vi "RS_SMBV100A_N_ASKCONFIGURATION.vi"(0 "DriverConnect in":T2={"InterfaceType"=enum."VISA", "OpenedSession"="", "InterfaceSettings"={"Interface"=enum."RS232", "EOS 4 read"=enum."LF (\\n)", "EOS 4 write"=enum."LF (\\n)", "TMO, ms"=10000, "Sett"=variant(cluster{"Baud Rate":u32, "Data Bits":u16, "Parity":u16, "Stop Bits":u16, "Flow Control":u16, "Eho":bool} {"Baud Rate"=75, "Data Bits"=0, "Parity"=0, "Stop Bits"=0, "Flow Control"=0, "Eho"=FALSE})}}, 1 "BASEBAND":string, 2 "mass":string, 9 "Error In":errorcluster) -> (3 "wrong sat":bool, 4 "DriverConnect out":T2={"InterfaceType"=enum."VISA", "OpenedSession"="", "InterfaceSettings"={"Interface"=enum."RS232", "EOS 4 read"=enum."LF (\\n)", "EOS 4 write"=enum."LF (\\n)", "TMO, ms"=10000, "Sett"=variant(cluster{"Baud Rate":u32, "Data Bits":u16, "Parity":u16, "Stop Bits":u16, "Flow Control":u16, "Eho":bool} {"Baud Rate"=75, "Data Bits"=0, "Parity"=0, "Stop Bits"=0, "Flow Control"=0, "Eho"=FALSE})}}, 6 "Parsing Satelite":T1, 10 "Error Out":errorcluster)   [LabVIEW 2018]
uses:
  MOKO_LabViewLibrary/MokoLowLevel/MokoLowLovelControl/MLLC_ConnectCluster.ctl
  MOKO_LabViewLibrary/MokoLowLevel/MokoLowLovelControl/MLLC_InterfaceType.ctl
  MOKO_LabViewLibrary/MokoLowLevel/MokoLowLovelControl/MLLC_OpenedSession.ctl
  MOKO_LabViewLibrary/MokoLowLevel/MokoLowLovelControl/MLLC_InterfaceSettings.ctl
  MOKO_LabViewLibrary/MokoLowLevel/MokoLowLovelControl/MLLC_InterfaceKind.ctl
  RS_SMBV100A_Parsing Satelite.ctl
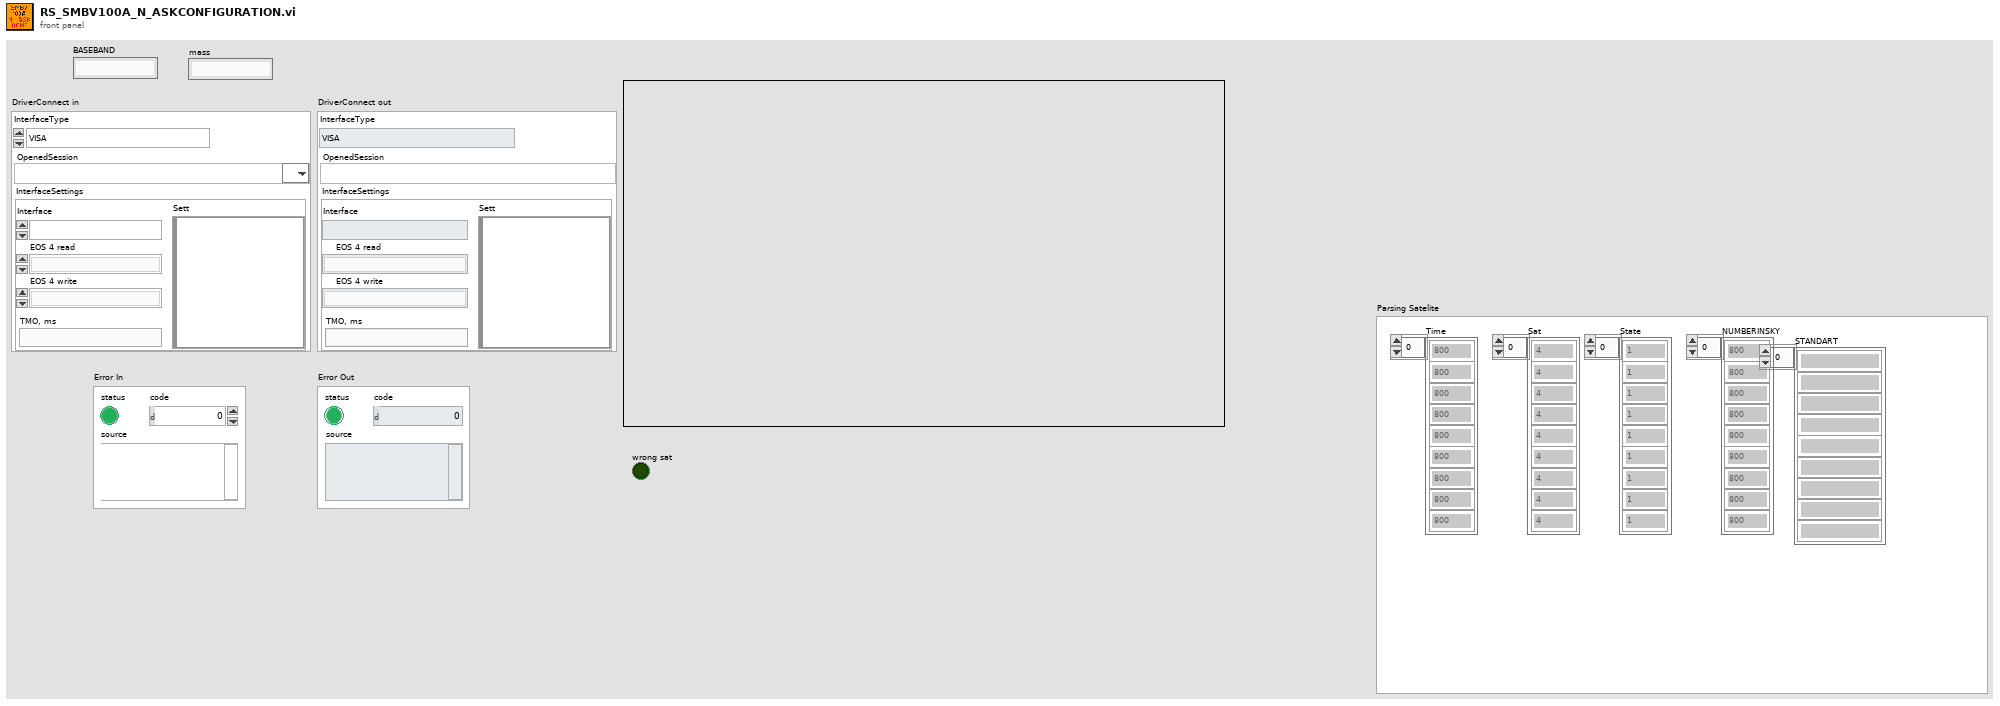
[diagram p1: front panel]
types:
  T1 = typedef "RS_SMBV100A_Parsing Satelite.ctl" = cluster{"Time":dbl[], "Sat":dbl[], "State":dbl[], "NUMBERINSKY":dbl[], "STANDART":string[]}
  T2 = typedef "MLLC_ConnectCluster.ctl" = cluster{"InterfaceType":T3, "OpenedSession":T4, "InterfaceSettings":T5}
  T3 = typedef "MLLC_InterfaceType.ctl" = enum16{"VISA", "Prologix USB-GPIB"}
  T4 = typedef "MLLC_OpenedSession.ctl" = refnum<visa-resource-name>
  T5 = typedef "MLLC_InterfaceSettings.ctl" = cluster{"Interface":T6, "EOS 4 read":enum16{"Default (=EOS 4 write)", "CR (\\r)", "LF (\\n)", "None"}, "EOS 4 write":enum16{"CR+LF (\\r\\n)", "CR (\\r)", "LF (\\n)", "None"}, "TMO, ms":i32, "Sett":variant}
  T6 = typedef "MLLC_InterfaceKind.ctl" = enum16{"RS232", "GPIB", "USB", "Ethernet", "another"}
  T7 = typedef "MLLC_Error.ctl" = errorcluster
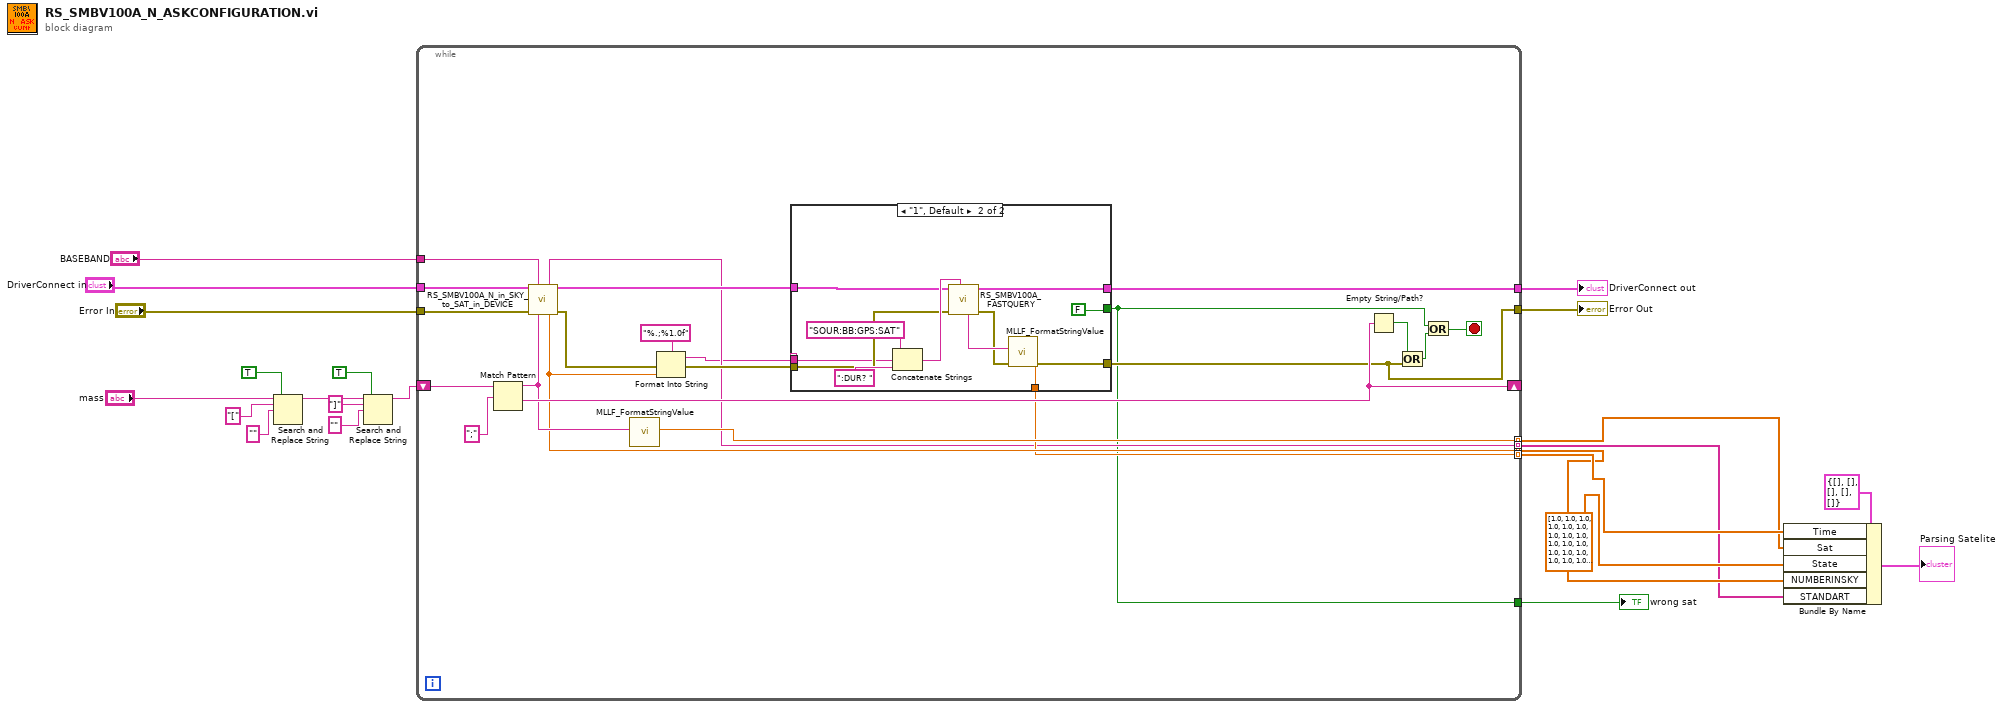
[diagram p0: block diagram]
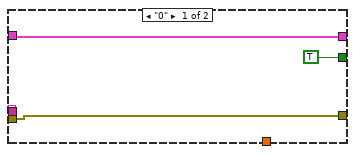
[diagram p2: hidden frame]
diagram:
  w6 = T1 {"Time"=[], "Sat"=[], "State"=[], "NUMBERINSKY"=[], "STANDART"=[]} ("Parsing Satelite")
  n1 = Search and Replace String(replace all?=TRUE, input string="mass", search string="[", replace string="") -> (result string=w15:string)  [unwired: 4 in, 3 out]
  n2 = Search and Replace String(replace all?=TRUE, input string=w15, search string="]", replace string="") -> (result string=w14:string)  [unwired: 4 in, 3 out]
  n3 = while {
    shift-right: [w41] -> _
    shift-left: w14 -> [w42]
    tunnel: [w36] -> w2 mode=indexing
    tunnel: [w39] -> w3 mode=indexing
    tunnel: [w34] -> w5 mode=indexing
    tunnel: "DriverConnect in" -> [w33]
    tunnel: "Error In" -> [w32]
    tunnel: [w31] -> w7
    tunnel: [w30] -> w1 mode=indexing
    tunnel: [w27] -> w9
    tunnel: "BASEBAND" -> [w26]
    tunnel: [w22] -> w11
    stop <- w24 stop-if-true
    n4 = Match Pattern(string=w42, regular expression=";") -> (before substring=w40:string, after substring=w41:string)  [unwired: 1 in, 2 out]
    n5 = call "RS_SMBV100A_N_in_SKY_to_SAT_in_DEVICE.vi"("DriverConnect in"=w33, "BASEBAND"=w26, "Error In"=w32, "String Value"=w40) -> ("GNSS"=w30:string, "DriverConnect out"=w35:T2, "SAT"=w36:dbl, "Error Out"=w29:errorcluster)  [unwired: 7 in, 1 out]
    n6 = call "MLLF_FormatStringValue.vi"("String Value"=w40) -> ("number"=w39:dbl)  [unwired: 8 in, 2 out]
    n7 = Format Into String(format string="%.;%1.0f" ("format"), error in=w29, w36) -> (resulting string=w23:string, error out=w37:errorcluster)  [unwired: 1 in]
    n8 = case shown="\"1\", Default" w23 {
      tunnel: w37 -> [w45 w53]
      tunnel: w23 -> [_ w52]
      tunnel: w35 -> [w46 w51]
      tunnel: [_ w50] -> w34
      tunnel: [w46 w49] -> w31
      tunnel: [w45 w48] -> w27
      tunnel: [TRUE FALSE] -> w22
      frame "0" {
      }
      frame "1", Default {
        n9 = Concatenate Strings("SOUR:BB:GPS:SAT" ("regular expression"), w52, ":DUR? " ("regular expression")) -> (w58:string)
        n10 = call "RS_SMBV100A_FASTQUERY.vi"("input"=w58, "Error In"=w53, "DriverConnect in"=w51) -> ("Error Out"=w54:errorcluster, "DriverConnect out"=w49:T2, "output"=w55:string)  [unwired: 6 in]
        n11 = call "MLLF_FormatStringValue.vi"("error in"=w54, "String Value"=w55) -> ("error out"=w48:T7, "number"=w50:dbl)  [unwired: 7 in, 1 out]
      }
    }
    n12 = Empty String/Path?(string/path=w41) -> (empty?=w28:bool)
    n13 = Or(x=w28, y=w27) -> (x .or. y?=w25:bool)
    n14 = Or(x=w22, y=w25) -> (x .or. y?=w24:bool)
  }
  "wrong sat" <- w11
  "Error Out" <- w9
  "DriverConnect out" <- w7
  n15 = Bundle By Name(cluster=w6, "Time"=w5, "Sat"=w3, "State"=dbl[] [1.0, 1.0, 1.0, 1.0, 1.0, 1.0, 1.0, 1.0, 1.0, 1.0, 1.0, 1.0, 1.0, 1.0, 1.0, 1.0, 1.0, 1.0, 1.0, 1.0, 1.0, 1.0, 1.0, 1.0, 1.0, 1.0, 1.0, 1.0, 1.0, 1.0, 1.0, 1.0, 1.0, 1.0, 1.0, 1.0, 1.0, 1.0, 1.0, 1.0, 1.0, 1.0, 1.0, 1.0, 1.0, 1.0, 1.0, 1.0, 1.0, 1.0, 1.0, 1.0], "NUMBERINSKY"=w2, "STANDART"=w1) -> ()  [unwired: 1 out]
  "Parsing Satelite" <- w6
